vi "Group_ToEasyObj.vi"(8 "error in (no error)":errorcluster, 11 "Group in":refnum<class "Group.lvclass">) -> (0 "error out":errorcluster, 2 "output cluster":T1 {"Channels"."Data Reference" format="%.0x"}, 3 "Group out":refnum<class "Group.lvclass">)   [LabVIEW 2023, in "Group.lvclass"]
doc: "Converts the group definition to a cluster definition from transferring between the System Explorer and Engine in VeriStand."
uses:
  Group.lvclass
  GroupAsCluster.ctl
  Channel/ChannelAsCluster.ctl
  <vilib>/NI VeriStand/Custom Device API/Data Reference.ctl
  Meta Data.ctl
  Group.lvclass/Group.ctl
  Channel/Channel.lvclass
  <vilib>/NI VeriStand/Custom Device API/Custom Device API.lvlib
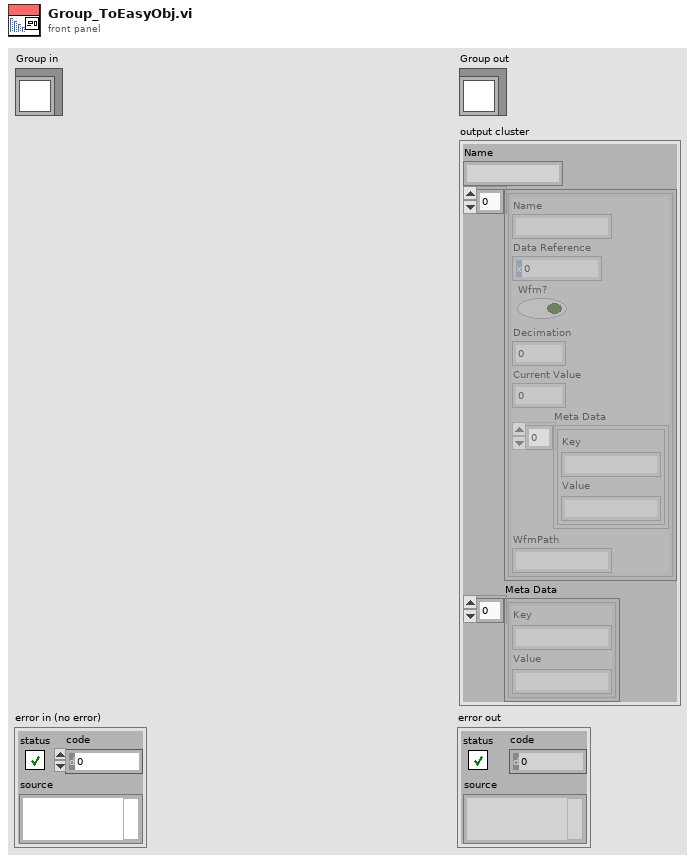
[diagram p1: front panel]
types:
  T1 = typedef "GroupAsCluster.ctl" = cluster{"Name":string, "Channels":T2[], "Meta Data":T4[]}
  T2 = typedef "ChannelAsCluster.ctl" = cluster{"Name":string, "Data Reference":T3, "Wfm?":bool, "Decimation":i32, "Current Value":dbl, "Meta Data":T4[], "WfmPath":string}
  T3 = typedef "Custom Device API.lvlib/Data Reference.ctl" = i32
  T4 = typedef "Meta Data.ctl" = cluster{"Key":string, "Value":string}
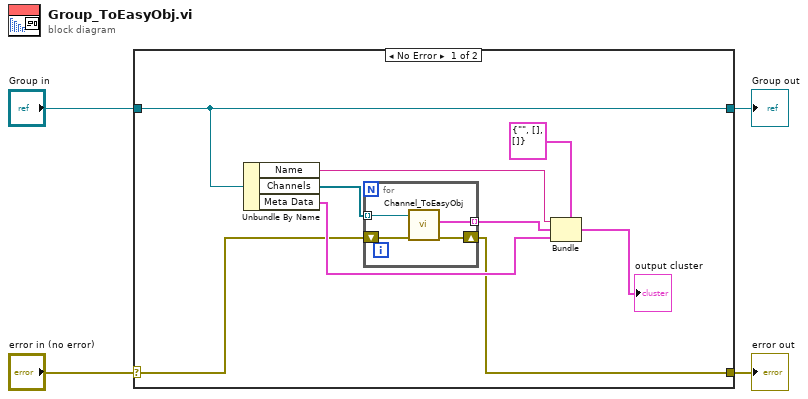
[diagram p0: block diagram]
diagram:
  n1 = case shown="No Error" "error in (no error)" {
    selector: "error in (no error)" -> [w6 w19]
    tunnel: [w5 w19] -> w3
    tunnel: [w7 w18] -> w1
    tunnel: "Group in" -> [w7 w18]
    frame No Error {
      n2 = Unbundle By Name(w7) -> ("Name"=w12:string, "Channels"=w13:refnum<class "Channel.lvclass">[], "Meta Data"=w10:T4[])
      n3 = for {
        tunnel: w13 -> [w17] mode=indexing
        tunnel: [w16] -> w11 mode=indexing
        shift-right: [w14] -> w5
        shift-left: w6 -> [w15]
        n4 = call-dynamic "Channel_ToEasyObj.vi"("error in (no error)"=w15, "Channel in"=w17) -> ("error out"=w14:errorcluster, "output cluster"=w16:T2)  [unwired: 7 in, 1 out]
      }
      n5 = Bundle(cluster=T1 {"Name"="", "Channels"=[], "Meta Data"=[]} ("output cluster"), "Name"=w12, "Channels"=w11, "Meta Data"=w10) -> (→"output cluster":T1)
    }
    frame Error {
    }
  }
  "error out" <- w3
  "Group out" <- w1
